vi "final polariser calib.vi"() -> ()   [LabVIEW 2017]
panel:
  out "Min Power":dbl
  out "Max Power":dbl
  out "Pos (M)":dbl
  out "Pos(m)":dbl
  out "Transmission Axis":dbl
  out "POWER":dbl[](array[numeric])
  out "POS":dbl[](array[numeric])
  out "Position":dbl[](array[numeric])
  out "Power":dbl[](array[numeric])
  in  "Flow Control(ms)":u32
  in  "STOP Program":bool
  in  "Milliseconds to wait":u32=1000
  in  "Axis in":i32=1
  out "Power vs Pos":cluster{"X":dbl[], "Y":dbl[]}[](graph) caption="XY Graph"
  in  "stop":bool
  out "Current Power":dbl format="%_4e"
  in  "Wavelength (nm)":u32=1064
  in  "VISA resource (In)":refnum<visa-resource-name>
  out "Curent pos (deg)":dbl format="%.2f"
  out "Initial pos (deg)":dbl format="%.2f"
  in  "SerialPort":u8=5
  # "Polariser Calibration"
  # "Motion control"
  # "Power control"
  # "Fine Tuning"
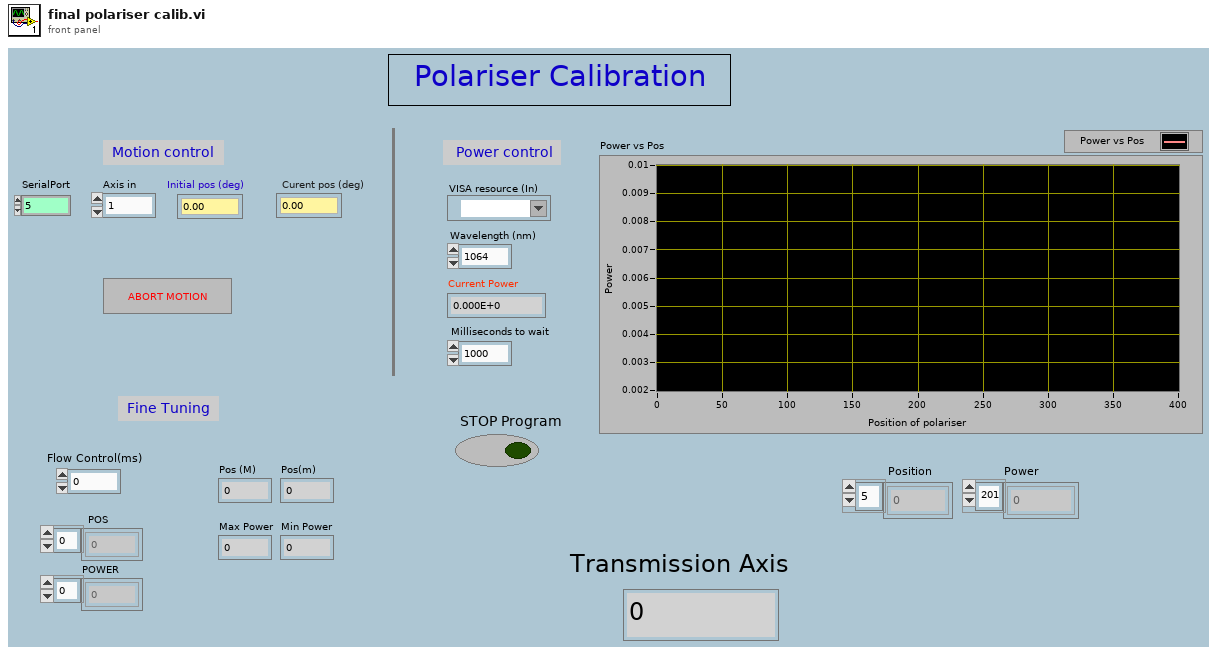
[diagram p1: front panel]
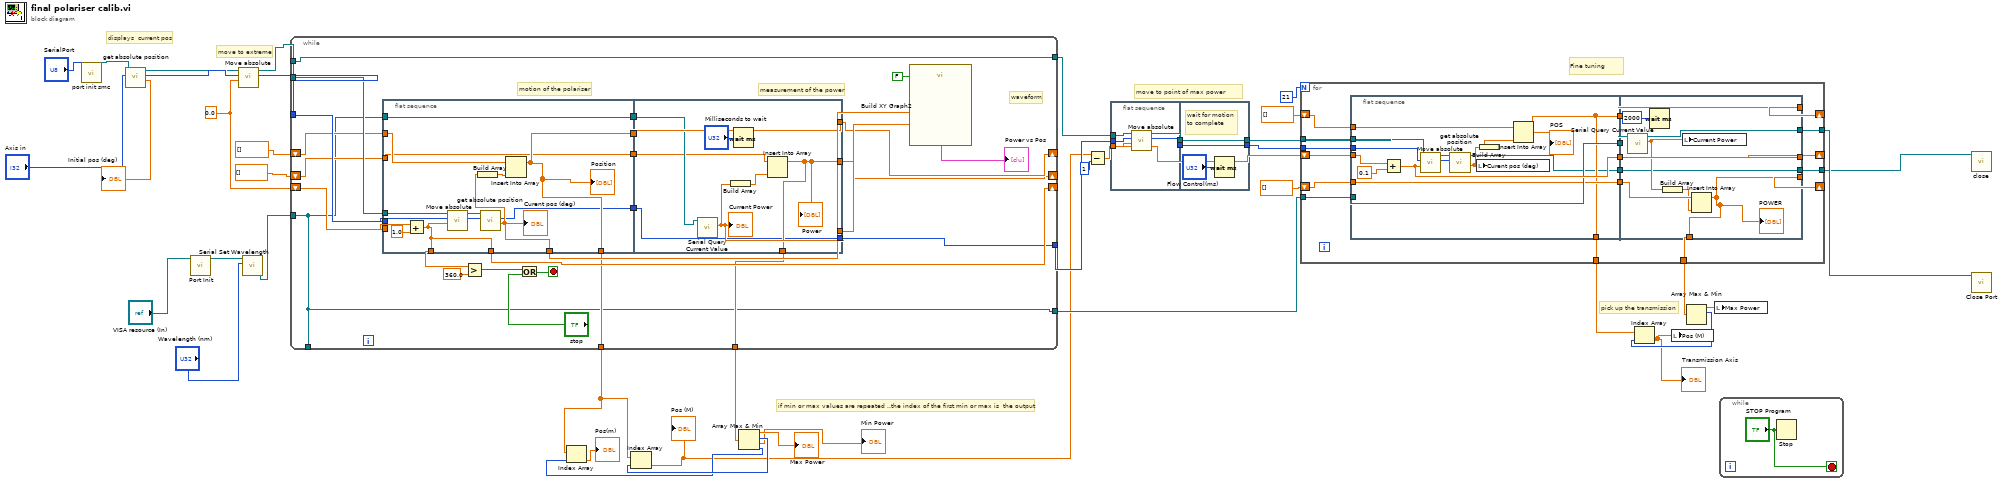
[diagram p0: block diagram]
diagram:
  w39 = 0.0 ("New target position (units)")
  # "pick up the transmission"
  # "move to point of max power"
  # "Fine tuning"
  # "if min or max values are repeated ..the index of the first min or max is  the output"
  # "move to extreme"
  # "displays  current pos"
  n1 = call <userlib>:"port init smc.vi"("SerialPort"="SerialPort") -> ("Visa Handle"=w37:refnum<visa-resource-name>)  [unwired: 3 in, 1 out]
  n2 = call <userlib>:"get absolute position.vi"("Axis in"="Axis in", "VISA Handle in"=w37) -> ("Target position (units)"=→"Initial pos (deg)":dbl, "Axis out"=w41:i32, "VISA Handle out"=w32:refnum<visa-resource-name>)  [unwired: 3 in, 2 out]
  n3 = call <instrlib>:"Port Init.vi"("VISA resource (In)"="VISA resource (In)") -> ("VISA resource (Out)"=w35:refnum<visa-resource-name>)  [unwired: 8 in, 2 out]
  n4 = call <userlib>:"Move absolute.vi"("New target position (units)"=w39, "Axis in"=w41, "VISA Handle in"=w32) -> ("Axis out"=w40:i32, "VISA Handle out"=w22:refnum<visa-resource-name>)  [unwired: 3 in, 2 out]
  n5 = call <instrlib>:"Serial Set Wavelength.vi"("Wavelength (nm)"="Wavelength (nm)", "VISA resource (In)"=w35) -> ("VISA resource (Out)"=w31:refnum<visa-resource-name>)  [unwired: 8 in, 1 out]
  n6 = while {
    tunnel: w22 -> [w68]
    tunnel: w40 -> [w67]
    shift-right: [w51] -> _
    shift-left: w39 -> [w66]
    tunnel: w31 -> [w47]
    tunnel: [w47] -> _
    tunnel: [w47] -> w19
    shift-right: [w54] -> _
    shift-left: dbl[] [] -> [w55]
    shift-right: [w52] -> _
    shift-left: dbl[] [] -> [w53]
    tunnel: [w50] -> w26
    tunnel: [w49] -> w24
    tunnel: [w45] -> w23
    tunnel: w22 -> [w44]
    tunnel: [w44] -> w20
    stop <- w59 stop-if-true
    # "waveform"
    # "measurement of the power"
    # "motion of the polariser"
    n7 = flat-sequence {
      tunnel: w68 -> [w82]
      tunnel: w67 -> [w81]
      tunnel: w66 -> [w78]
      tunnel: [w76] -> w65
      tunnel: [w74] -> w60
      tunnel: [w73] -> w56
      tunnel: w55 -> [w70]
      tunnel: w53 -> [w69]
      tunnel: [w74] -> w51
      tunnel: [w73] -> w49
      tunnel: [w72] -> w48
      tunnel: w47 -> [w72]
      tunnel: [w71] -> w46
      tunnel: [w69] -> w43
      tunnel: [w88] -> w58
      tunnel: w56 -> [w89]
      tunnel: [w89] -> w54
      tunnel: [w86] -> w52
      tunnel: [w86] -> w50
      tunnel: w48 -> [w85]
      tunnel: w46 -> [w84]
      tunnel: [w84] -> w45
      tunnel: w43 -> [w83]
      frame #0 {
        n8 = Add(x=w78, y=1.0) -> (x+y=w74:dbl)
        n9 = call <userlib>:"Move absolute.vi"("New target position (units)"=w74, "Axis in"=w81, "VISA Handle in"=w82) -> ("Axis out"=w79:i32, "VISA Handle out"=w80:refnum<visa-resource-name>)  [unwired: 3 in, 2 out]
        n10 = call <userlib>:"get absolute position.vi"("Axis in"=w79, "VISA Handle in"=w80) -> ("Target position (units)"=w76:dbl, "Axis out"=w71:i32)  [unwired: 3 in, 3 out]
        "Curent pos (deg)" <- w76
        n11 = Build Array(w76) -> (w75:dbl[])
        n12 = Insert Into Array(array=w70, new element=w75) -> (w73:dbl[])  [unwired: 1 in]
        "Position" <- w73
      }
      frame #1 {
        n13 = call <instrlib>:"Serial Query Current Value.vi"("VISA resource (In)"=w85) -> ("Current Value"=w88:dbl)  [unwired: 8 in, 2 out]
        "Current Power" <- w88
        n14 = Build Array(w88) -> (w87:dbl[])
        n15 = Wait (ms)(milliseconds to wait="Milliseconds to wait") -> ()  [unwired: 1 out]
        n16 = Insert Into Array(array=w83, new element=w87) -> (w86:dbl[])  [unwired: 1 in]
        "Power" <- w86
      }
    }
    n17 = Greater?(x=w60, y=360.0) -> (0:w62:bool)
    n18 = Or(x=w62, y="stop") -> (x .or. y?=w59:bool)
    n19 = call "Build XY Graph2"("Reset"=FALSE, "Y Input"=w58, "X Input"=w65) -> ("XY Graph"=→"Power vs Pos":cluster{"X":dbl[], "Y":dbl[]}[])  [unwired: 7 in, 1 out]
  }
  n20 = Array Max & Min(array=w26) -> (max value=→"Max Power":dbl, max index (indices)=w33:i32, min value=→"Min Power":dbl, min index (indices)=w29:i32)
  n21 = Index Array(array=w24, index=w29) -> (element=→"Pos(m)":dbl)
  n22 = Index Array(array=w24, index=w33) -> (element=w18:dbl)
  "Pos (M)" <- w18
  n23 = Subtract(x=w18, y=1) -> (x-y=w15:dbl)
  n24 = flat-sequence {
    tunnel: w23 -> [w95]
    tunnel: w20 -> [w93]
    tunnel: w15 -> [w91]
    tunnel: [w94] -> w13
    tunnel: [w92] -> w12
    tunnel: [w97] -> w16
    tunnel: [w98] -> w21
    tunnel: w13 -> [w98]
    tunnel: w12 -> [w97]
    frame #0 {
      n25 = call <userlib>:"Move absolute.vi"("New target position (units)"=w91, "Axis in"=w95, "VISA Handle in"=w93) -> ("Axis out"=w92:i32, "VISA Handle out"=w94:refnum<visa-resource-name>)  [unwired: 3 in, 2 out]
    }
    frame #1 {
      # "wait for motion\nto complete"
      n26 = Wait (ms)(milliseconds to wait="Flow Control(ms)") -> ()  [unwired: 1 out]
    }
  }
  n27 = for {
    N: 21 -> [_]
    tunnel: w21 -> [w115]
    shift-right: [w114] -> _
    shift-left: w15 -> [w116]
    tunnel: w19 -> [w111]
    tunnel: w16 -> [w110]
    shift-right: [w104] -> _
    shift-left: dbl[] [] -> [w107]
    shift-right: [w105] -> _
    shift-left: dbl[] [] -> [w109]
    tunnel: [w103] -> w9
    tunnel: [w102] -> w8
    tunnel: [w101] -> w6
    tunnel: [w99] -> w5
    n28 = flat-sequence {
      tunnel: w116 -> [w129]
      tunnel: w115 -> [w128]
      tunnel: [w127] -> w113
      tunnel: [w126] -> w112
      tunnel: w111 -> [w126]
      tunnel: w110 -> [w125]
      tunnel: w109 -> [w120]
      tunnel: [w119] -> w108
      tunnel: w107 -> [w119]
      tunnel: [w118] -> w106
      tunnel: [w118] -> w102
      tunnel: [w117] -> w100
      tunnel: [w140] -> w114
      tunnel: w113 -> [w140]
      tunnel: w112 -> [w138]
      tunnel: w108 -> [w135]
      tunnel: [w137] -> w105
      tunnel: w106 -> [w137]
      tunnel: [w133] -> w104
      tunnel: [w133] -> w103
      tunnel: [w132] -> w101
      tunnel: w100 -> [w131]
      tunnel: [w131] -> w99
      frame #0 {
        n29 = Add(x=w129, y=0.1) -> (x+y=w127:dbl)
        n30 = call <userlib>:"Move absolute.vi"("New target position (units)"=w127, "Axis in"=w125, "VISA Handle in"=w128) -> ("Axis out"=w124:i32, "VISA Handle out"=w123:refnum<visa-resource-name>)  [unwired: 3 in, 2 out]
        n31 = call <userlib>:"get absolute position.vi"("Axis in"=w124, "VISA Handle in"=w123) -> ("Target position (units)"=w122:dbl, "VISA Handle out"=w117:refnum<visa-resource-name>)  [unwired: 3 in, 3 out]
        n32 = local write "Curent pos (deg)"(w122) -> ()
        n33 = Build Array(w122) -> (w121:dbl[])
        n34 = Insert Into Array(array=w120, new element=w121) -> (w118:dbl[])  [unwired: 1 in]
        "POS" <- w118
      }
      frame #1 {
        n35 = call <instrlib>:"Serial Query Current Value.vi"("VISA resource (In)"=w138) -> ("Current Value"=w136:dbl, "VISA resource (Out)"=w132:refnum<visa-resource-name>)  [unwired: 8 in, 1 out]
        n36 = Wait (ms)(milliseconds to wait=u32 2000) -> ()  [unwired: 1 out]
        n37 = Build Array(w136) -> (w134:dbl[])
        n38 = local write "Current Power"(w136) -> ()
        n39 = Insert Into Array(array=w135, new element=w134) -> (w133:dbl[])  [unwired: 1 in]
        "POWER" <- w133
      }
    }
  }
  n40 = Array Max & Min(array=w9) -> (max value=w2:dbl, max index (indices)=w7:i32)  [unwired: 2 out]
  n41 = Index Array(array=w8, index=w7) -> (element=w1:dbl)
  "Transmission Axis" <- w1
  n42 = local write "Pos (M)"(w1) -> ()
  n43 = local write "Max Power"(w2) -> ()
  n44 = while {
    stop <- "STOP Program" stop-if-true
    n45 = Stop(stop? (T)="STOP Program") -> ()
  }
  n46 = call <userlib>:"close.vi"("VISA Handle in"=w5) -> ()  [unwired: 4 in, 1 out]
  n47 = call <instrlib>:"Close Port.vi"("VISA resource (In)"=w6) -> ()  [unwired: 10 in, 1 out]
